vi "New Camera Selection.vi"(8 "error in (no error)":errorcluster, 10 "New Camera Selection":string, 11 "HIJ Vision Camera App Dialog in":refnum<class "HIJ Vision Camera App Dialog.lvclass">) -> (0 "error out":errorcluster, 3 "HIJ Vision Camera App Dialog out":refnum<class "HIJ Vision Camera App Dialog.lvclass">)   [LabVIEW 2014, in "HIJ Vision Camera App Dialog.lvlib" / "HIJ Vision Camera App Dialog.lvclass"]
uses:
  HIJ Vision Camera App Dialog.lvclass
  HIJ Vision Camera App Dialog.lvclass/HIJ Vision Camera App Dialog.ctl
  Shared Code/Viewable Actor/ViewableActor/ViewableActor.lvclass
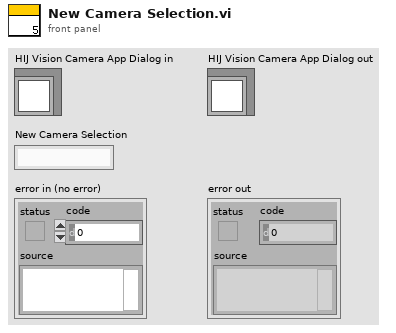
[diagram p1: front panel]
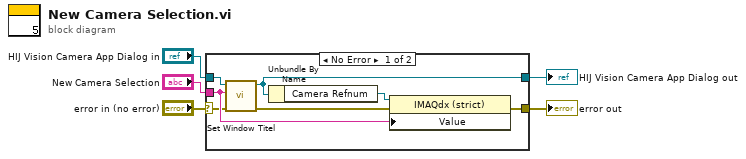
[diagram p0: block diagram]
diagram:
  n1 = case shown="No Error" "error in (no error)" {
    selector: "error in (no error)" -> [w7 w14]
    tunnel: [w10 w14] -> w4
    tunnel: [w9 w13] -> w2
    tunnel: "HIJ Vision Camera App Dialog in" -> [w12 w13]
    tunnel: "New Camera Selection" -> [w8 _]
    frame No Error {
      n2 = call "Set Window Titel.vi"("error in (no error)"=w7, "Title"=w8, "ViewableActor in"=w12) -> ("error out"=w6:errorcluster, "ViewableActor out"=w9:refnum<class "HIJ Vision Camera App Dialog.lvclass">)  [unwired: 7 in]
      n3 = Unbundle By Name(w9) -> ("Camera Refnum"=w11:refnum<vi>)
      n4 = property class="IMAQdx (strict)"(reference=w11, error in=w6, "Value"=w8) -> (error out=w10:errorcluster)  [unwired: 1 out]
    }
    frame Error {
    }
  }
  "error out" <- w4
  "HIJ Vision Camera App Dialog out" <- w2
